vi "Lake Shore Cryotronics 331 Application Temperature Controller.vi"(1 "Loop (0: 1)":u16(ring) items=["1", "2"], 2 "Gain (P) (0.0)":dbl min=0.0 max=1000.0 step=0.1 format="%.1f", 3 "Reset (I) (0.0)":dbl min=0.0 max=1000.0 step=0.1 format="%.1f", 4 "Rate (D) (0)":dbl min=0.0 max=200.0 step=1.0, 6 "Configure (False)":bool, 7 "Manual Output (0.000)":dbl min=0.0 max=100.0 step=0.001 format="%.3f", 8 "Input (0: A)":u16(ring) items=["A", "B"], 9 "Heater Range (0: Off)":u16(ring) items=["Off", "Low (0.5W)", "Med (5W)", "High (50W)"], 11 "Setpoint (0.0000)":dbl min=-273.0 max=300000.0 step=0.0001 format="%.4f") -> (15 "Celsius Reading":dbl min=-273.16 max=1372.0 step=1e-05 format="%^.5e", 16 "Kelvin Reading":dbl min=0.0 max=1645.0 step=1e-05 format="%^.5e", 17 "Sensor Units Reading":dbl min=-7.5 max=300000.0 step=1e-05 format="%^.5e", 18 "Loop 1\nHeater Output":dbl(slide) min=0.0 max=100.0 step=0.01 scale=0.0..100.0 scale format="%.1f")   [LabVIEW 2010]
doc: "This VI was designed to demonstrate typical usage of sub vi's containing the more common 331 functions.\n\nThis example configures the loop and setpoint of the instrument, allows for a delay, and then reads sensor and heater output data. The user is given the option of just reading data and not configuring the instrument."
uses:
  <instrlib>/Lake Shore Cryotronics 331/Lake Shore Cryotronics 331.lvlib
panel:
  in  "VISA resource name":refnum<visa-resource-name>
  # "(c) 2007-2009 Lake Shore Cryotronics Inc.  ALL RIGHTS RESERVED."
  # "%"
  # "331 Temperature Controller"
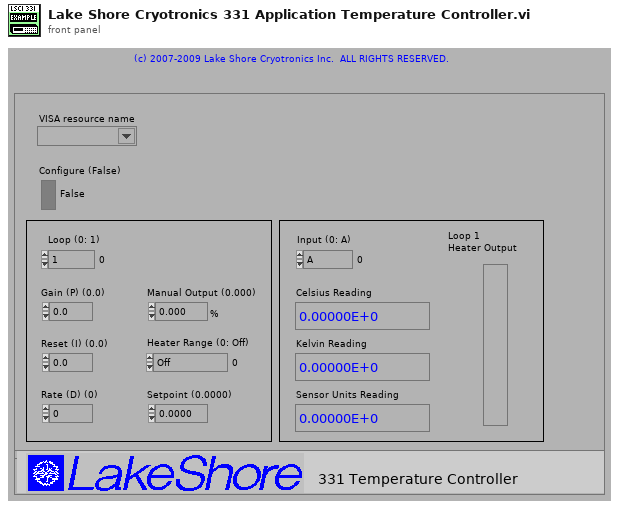
[diagram p1: front panel]
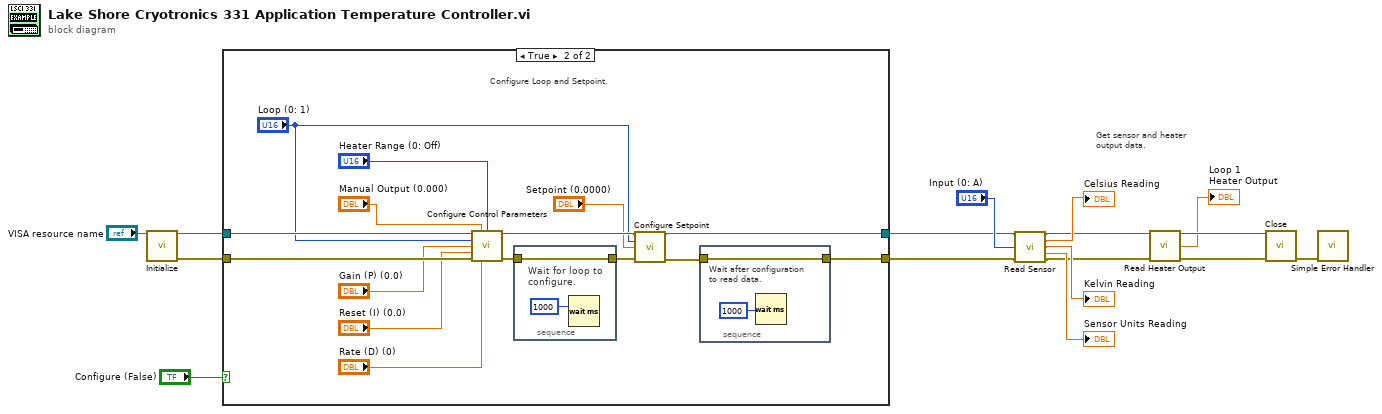
[diagram p0: block diagram]
diagram:
  # "Get sensor and heater\noutput data."
  n1 = call <instrlib>:"Initialize.vi"("VISA resource name"="VISA resource name") -> ("VISA resource name out"=w14:refnum<visa-resource-name>, "error out"=w13:errorcluster)  [unwired: 13 in]
  n2 = case shown="True" "Configure (False)" {
    tunnel: w13 -> [w17 w30]
    tunnel: w14 -> [w18 w31]
    tunnel: [w17 w33] -> w9
    tunnel: [w18 w22] -> w10
    frame False {
      # "Do not configure Loop and Setpoint."
    }
    frame True {
      # "Configure Loop and Setpoint."
      n3 = call <instrlib>:"Configure Control Parameters.vi"("VISA resource name"=w31, "Manual Output (0.000 %)"="Manual Output (0.000)", "Heater Range (0: Off)"="Heater Range (0: Off)", "Loop (0: 1)"="Loop (0: 1)", "Gain (P) (0.0)"="Gain (P) (0.0)", "Reset (I) (0.0)"="Reset (I) (0.0)", "error in (no error)"=w30, "Rate (D) (0)"="Rate (D) (0)") -> ("VISA resource name out"=w21:refnum<visa-resource-name>, "error out"=w32:errorcluster)  [unwired: 6 in]
      n4 = stacked-sequence {
        tunnel: w32 -> [w36]
        tunnel: [w36] -> w24
        frame #0 {
          # "Wait for loop to \nconfigure."
          n5 = Wait (ms)(milliseconds to wait=u32 1000) -> ()  [unwired: 1 out]
        }
      }
      n6 = call <instrlib>:"Configure Setpoint.vi"("VISA resource name"=w21, "Loop (0: 1)"="Loop (0: 1)", "Setpoint (0.0000)"="Setpoint (0.0000)", "error in (no error)"=w24) -> ("VISA resource name out"=w22:refnum<visa-resource-name>, "error out"=w23:errorcluster)  [unwired: 10 in]
      n7 = stacked-sequence {
        tunnel: w23 -> [w35]
        tunnel: [w35] -> w33
        frame #0 {
          # "Wait after configuration\nto read data."
          n8 = Wait (ms)(milliseconds to wait=1000) -> ()  [unwired: 1 out]
        }
      }
    }
  }
  n9 = call <instrlib>:"Read Sensor.vi"("VISA resource name"=w10, "Input (0: A)"="Input (0: A)", "error in (no error)"=w9) -> ("VISA resource name out"=w5:refnum<visa-resource-name>, "Celsius Reading"=→"Celsius Reading":dbl, "Kelvin Reading"=→"Kelvin Reading":dbl, "Sensor Units Reading"=→"Sensor Units Reading":dbl, "error out"=w4:errorcluster)  [unwired: 8 in]
  n10 = call <instrlib>:"Read Heater Output.vi"("VISA resource name"=w5, "error in (no error)"=w4) -> ("VISA resource name out"=w2:refnum<visa-resource-name>, "Loop 1\nHeater Output"=→"Loop 1\nHeater Output":dbl, "error out"=w3:errorcluster)  [unwired: 11 in]
  n11 = call <instrlib>:"Close.vi"("VISA resource name"=w2, "error in (no error)"=w3) -> ("error out"=w15:errorcluster)  [unwired: 13 in]
  n12 = call <vilib>:"Simple Error Handler.vi"("error in (no error)"=w15) -> ()  [unwired: 4 in, 5 out]
